vi "TstBldr_AnalysisScripts.vi"(0 "Engine reference":refnum<k7>, 1 "paths":T1, 2 "First call?":bool=TRUE, 5 "Sequence File Ref":refnum<k7>, 7 "Step Name":string="Run Script", 9 "Requirement":string, 11 "error in":errorcluster, 12 "Sequence index":i32, 13 "Conition Run?":bool, 14 "Attended?":bool) -> (3 "First call? out":bool, 4 "Engine reference (out)":refnum<k7>, 6 "Sequence File Ref(out)":refnum<k7>, 8 "Sequence index (out)":i32, 15 "error out":errorcluster)   [LabVIEW 2010]
doc: "This VI creates steps in TestStand for running analysis scripts in DIAdem"
uses:
  FilePaths.ctl
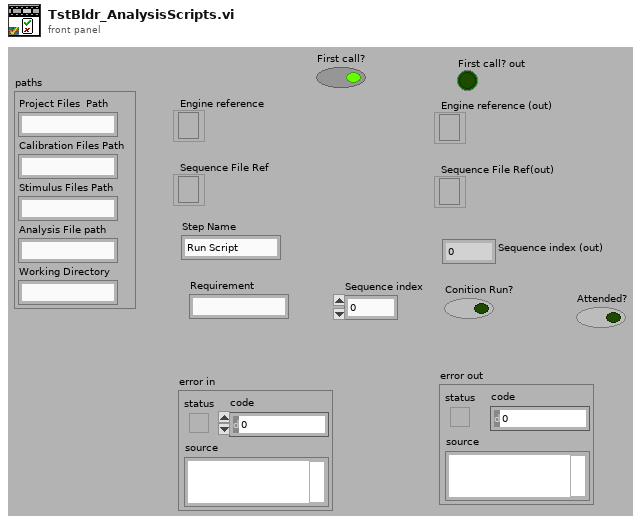
[diagram p1: front panel]
types:
  T1 = typedef "FilePaths.ctl" = cluster{"Project Files  Path":string, "Calibration Files Path":string, "Stimulus Files Path":string, "Analysis File path":string, "Working Directory":string}
  T2 = enum16{"Open DD Ref", "Export Paths", "Run Script", "Import Results", "Analysis Results", "Close DD Ref"}
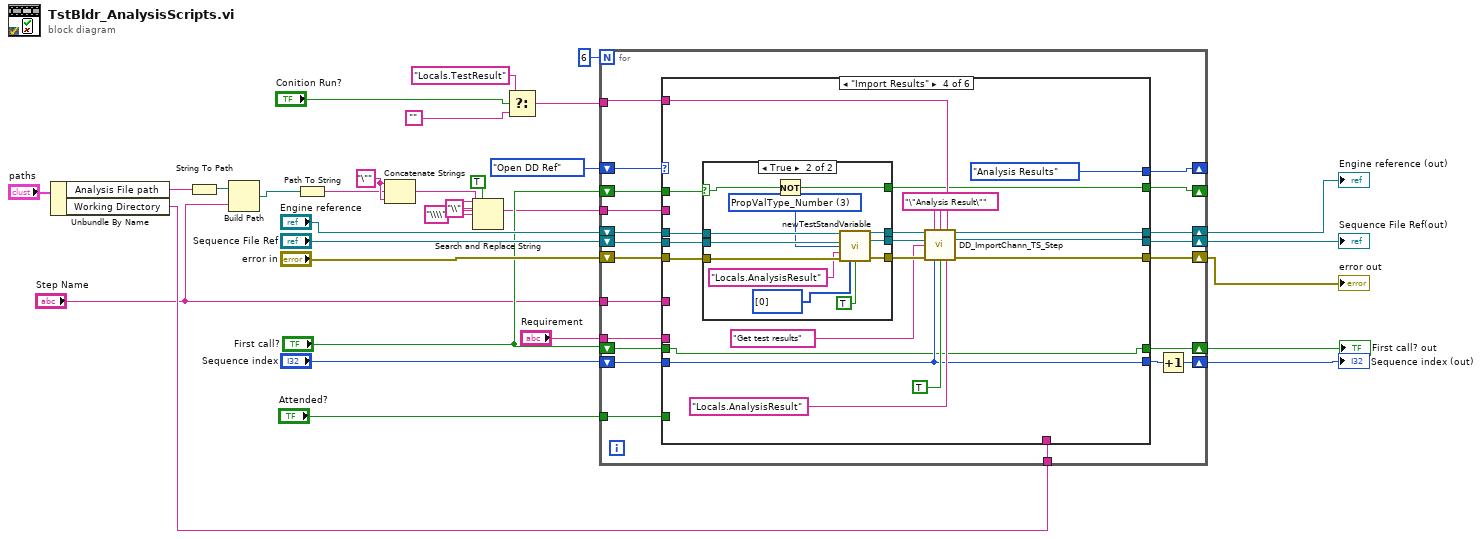
[diagram p0: block diagram]
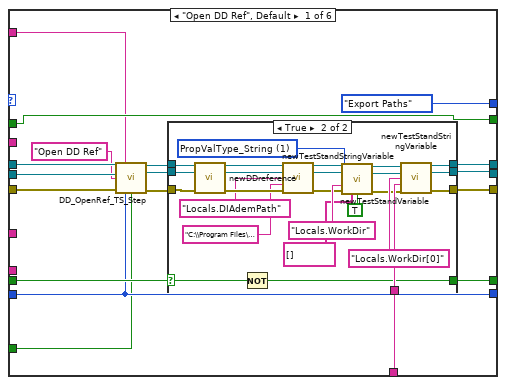
[diagram p2: hidden frame]
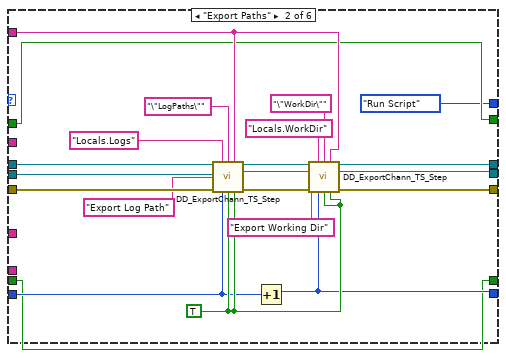
[diagram p4: hidden frame]
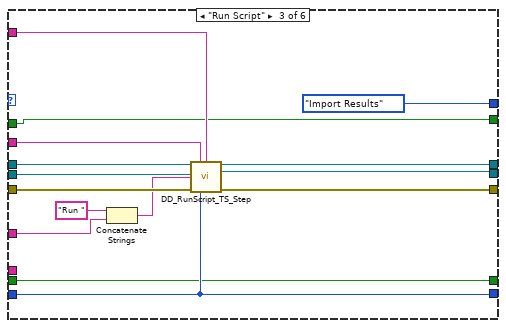
[diagram p5: hidden frame]
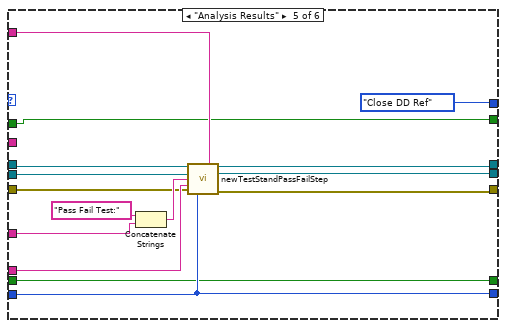
[diagram p7: hidden frame]
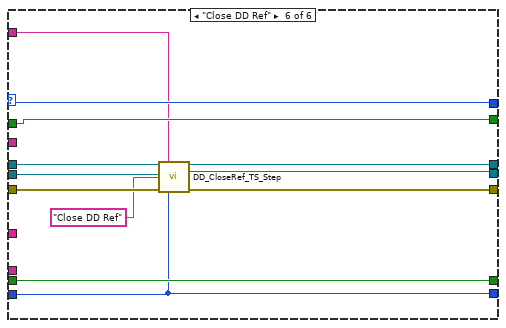
[diagram p8: hidden frame]
diagram:
  w11 = "\"" ("string")
  n1 = Unbundle By Name("paths") -> ("Analysis File path"=w5:string, "Working Directory"=w6:string)
  n2 = String To Path(string=w5) -> (path=w4:path)
  n3 = Build Path(base path=w4, name or relative path="Step Name") -> (appended path=w2:path)
  n4 = Path To String(path=w2) -> (string=w1:string)
  n5 = Concatenate Strings(w11, w1, w11) -> (w15:string)
  n6 = Search and Replace String(replace all?=TRUE ("replace all? (F)"), input string=w15, search string="\\", replace string="\\\\" ("replace string (\"\")")) -> (result string=w10:string)  [unwired: 4 in, 3 out]
  n7 = Select(t="Locals.TestResult", s="Conition Run?", f="") -> (s? t:f=w18:string)
  n8 = for {
    N: 6 -> [_]
    shift-right: [w48] -> w28
    shift-left: "Engine reference" -> [w51]
    shift-right: [w47] -> w29
    shift-left: "Sequence File Ref" -> [w50]
    shift-right: [w46] -> w30
    shift-left: "error in" -> [w49]
    shift-right: [w45] -> _
    shift-left: T2."Open DD Ref" -> [w52]
    tunnel: "Step Name" -> [w44]
    tunnel: w10 -> [w43]
    tunnel: "Requirement" -> [w41]
    tunnel: w6 -> [w40]
    shift-right: [w38] -> w31
    shift-left: "Sequence index" -> [w39]
    tunnel: w18 -> [w37]
    shift-right: [w35] -> w17
    shift-left: "First call?" -> [w36]
    shift-right: [w33] -> _
    shift-left: "First call?" -> [w34]
    tunnel: "Attended?" -> [w32]
    n9 = case shown="\"Import Results\"" w52 {
      selector: w52 -> [_ _ _ _ _ w188]
      tunnel: w51 -> [w60 w120 w135 w155 w186 w192]
      tunnel: w50 -> [w59 w119 w134 w154 w185 w191]
      tunnel: w49 -> [w63 w121 w136 w153 w172 w196]
      tunnel: [w70 w112 w132 w147 w184 w193] -> w48
      tunnel: [w69 w111 w130 w148 w183 w194] -> w47
      tunnel: [w68 w110 w131 w149 w182 w195] -> w46
      tunnel: [T2."Export Paths" T2."Run Script" T2."Import Results" T2."Analysis Results" T2."Close DD Ref" w188] -> w45
      tunnel: w39 -> [w58 w105 w129 w142 w181 w189]
      tunnel: w44 -> [_ _ w127 _ w178 _]
      tunnel: w43 -> [_ _ w133 _ _ _]
      tunnel: [w58 w104 w129 w142 w181 w189] -> w42
      tunnel: w41 -> [_ _ _ _ w180 _]
      tunnel: w40 -> [w67 _ _ _ _ _]
      tunnel: w37 -> [w53 w103 w125 w141 w176 w187]
      tunnel: w36 -> [w66 w102 w124 w140 w175 w198]
      tunnel: [w65 w102 w124 w140 w175 w198] -> w35
      tunnel: w34 -> [w64 w101 w123 w139 w174 w197]
      tunnel: [w64 w101 w123 w138 w174 w197] -> w33
      tunnel: w32 -> [w56 _ _ _ _ _]
      frame "Open DD Ref", Default {
        n10 = call "DD_OpenRef_TS_Step.vi"("Engine Reference"=w60, "Precondition"=w53, "Sequence File Ref"=w59, "Step Name"="Open DD Ref", "error in"=w63, "index"=w58, "Attended?"=w56) -> ("Engine reference(out)"=w62:refnum<k7>, "Sequence File Ref(out)"=w61:refnum<k7>, "error out"=w55:errorcluster)  [unwired: 6 in]
        n11 = case shown="True" w66 {
          selector: w66 -> [w71 w89]
          tunnel: w62 -> [w74 w85]
          tunnel: w61 -> [w73 w86]
          tunnel: w55 -> [w72 w87]
          tunnel: [w74 w99] -> w70
          tunnel: [w73 w98] -> w69
          tunnel: [w72 w97] -> w68
          tunnel: w67 -> [_ w95]
          tunnel: [w71 w88] -> w65
          frame False {
          }
          frame True {
            w91 = 1 items=["PropValType_Container", "PropValType_String", "PropValType_Boolean", "PropValType_Number", "PropValType_NamedType", "PropValType_Reference", "PropValType_Array"] ("Variable Type")
            n12 = call "newDDreference.vi"("Engine Reference"=w85, "Sequence File Ref"=w86, "error in"=w87) -> ("Engine Reference (out)"=w80:refnum<k7>, "Sequence File (out)"=w79:refnum<k7>, "error out"=w84:errorcluster)  [unwired: 10 in]
            n13 = Not(x=w89) -> (.not. x?=w88:bool)
            n14 = call "newTestStandStringVariable.vi"("Engine Reference"=w80, "Sequence File Ref"=w79, "Variable Name"="Locals.DIAdemPath", "Variable Value"="C:\\Program Files\\National Instruments\\DIAdem 11.1", "error in"=w84) -> ("Engine Reference (out)"=w82:refnum<k7>, "Sequence File (out)"=w81:refnum<k7>, "error out"=w83:errorcluster)  [unwired: 8 in]
            n15 = call "newTestStandVariable.vi"("Engine Reference"=w82, "Sequence File Ref"=w81, "Variable Type"=w91, "Variable Name"="Locals.WorkDir", "error in"=w83, "Variable Value"=string[] [], "Array?"=TRUE) -> ("Engine Reference(out)"=w93:refnum<k7>, "Sequence File Ref(out)"=w92:refnum<k7>, "error out"=w94:errorcluster)  [unwired: 6 in]
            n16 = call "newTestStandStringVariable.vi"("Engine Reference"=w93, "Sequence File Ref"=w92, "Variable Name"="Locals.WorkDir[0]", "Variable Value"=w95, "error in"=w94) -> ("Engine Reference (out)"=w99:refnum<k7>, "Sequence File (out)"=w98:refnum<k7>, "error out"=w97:errorcluster)  [unwired: 8 in]
          }
        }
      }
      frame "Export Paths" {
        w106 = TRUE ("Use Name?")
        n17 = call "DD_ExportChann_TS_Step.vi"("Engine Reference"=w120, "Source Data"="Locals.Logs", "Channel Name"="\"LogPaths\"", "Precondition"=w103, "Sequence File Ref"=w119, "Step Name"="Export Log Path", "error in"=w121, "index"=w105, "Use Name?"=w106, "CreateChannel?"=w106) -> ("Engine reference(out)"=w115:refnum<k7>, "Sequence File Ref(out)"=w113:refnum<k7>, "error out"=w114:errorcluster)  [unwired: 3 in]
        n18 = Increment(x=w105) -> (x+1=w104:i32)
        n19 = call "DD_ExportChann_TS_Step.vi"("Engine Reference"=w115, "Source Data"="Locals.WorkDir", "Channel Name"="\"WorkDir\"", "Precondition"=w103, "Sequence File Ref"=w113, "Step Name"="Export Working Dir", "error in"=w114, "index"=w104, "Use Name?"=w106, "CreateChannel?"=w106) -> ("Engine reference(out)"=w112:refnum<k7>, "Sequence File Ref(out)"=w111:refnum<k7>, "error out"=w110:errorcluster)  [unwired: 3 in]
      }
      frame "Run Script" {
        n20 = Concatenate Strings("Run " ("Step Name"), w127) -> (w126:string)
        n21 = call "DD_RunScript_TS_Step.vi"("Engine Reference"=w135, "Script Path"=w133, "Precondition"=w125, "Sequence File Ref"=w134, "Step Name"=w126, "error in"=w136, "index"=w129) -> ("Engine reference(out)"=w132:refnum<k7>, "Sequence File Ref(out)"=w130:refnum<k7>, "error out"=w131:errorcluster)  [unwired: 6 in]
      }
      frame "Import Results" {
        w145 = "\"Analysis Result\"" ("FirstChannel")
        n22 = case shown="True" w139 {
          selector: w139 -> [w156 w163]
          tunnel: w155 -> [w159 w171]
          tunnel: w154 -> [w158 w170]
          tunnel: w153 -> [w157 w169]
          tunnel: [w159 w166] -> w152
          tunnel: [w158 w165] -> w151
          tunnel: [w157 w164] -> w150
          tunnel: [w156 w162] -> w138
          frame False {
          }
          frame True {
            w168 = 3 items=["PropValType_Container", "PropValType_String", "PropValType_Boolean", "PropValType_Number", "PropValType_NamedType", "PropValType_Reference", "PropValType_Array"] ("Variable Type")
            n23 = Not(x=w163) -> (.not. x?=w162:bool)
            n24 = call "newTestStandVariable.vi"("Engine Reference"=w171, "Sequence File Ref"=w170, "Variable Type"=w168, "Variable Name"="Locals.AnalysisResult", "error in"=w169, "Variable Value"=i32[] [0], "Array?"=TRUE) -> ("Engine Reference(out)"=w166:refnum<k7>, "Sequence File Ref(out)"=w165:refnum<k7>, "error out"=w164:errorcluster)  [unwired: 6 in]
          }
        }
        n25 = call "DD_ImportChann_TS_Step.vi"("Engine Reference"=w152, "FirstChannel"=w145, "LastChannel"=w145, "Precondition"=w141, "Sequence File Ref"=w151, "Step Name"="Get test results", "error in"=w150, "index"=w142, "Use Name?"=TRUE, "Data Output"="Locals.AnalysisResult") -> ("Engine reference(out)"=w147:refnum<k7>, "Sequence File Ref(out)"=w148:refnum<k7>, "error out"=w149:errorcluster)  [unwired: 3 in]
      }
      frame "Analysis Results" {
        n26 = Concatenate Strings("Pass Fail Test:" ("Step Name"), w178) -> (w177:string)
        n27 = call "newTestStandPassFailStep.vi"("Engine Reference"=w186, "Precondition"=w176, "Sequence File Ref"=w185, "Step Name"=w177, "Requirement"=w180, "error in"=w172, "index"=w181) -> ("Engine reference(out)"=w184:refnum<k7>, "Sequence File Ref(out)"=w183:refnum<k7>, "error out"=w182:errorcluster)  [unwired: 6 in]
      }
      frame "Close DD Ref" {
        n28 = call "DD_CloseRef_TS_Step.vi"("Engine Reference"=w192, "Precondition"=w187, "Sequence File Ref"=w191, "Step Name"="Close DD Ref", "error in"=w196, "index"=w189) -> ("Engine reference(out)"=w193:refnum<k7>, "Sequence File Ref(out)"=w194:refnum<k7>, "error out"=w195:errorcluster)  [unwired: 7 in]
      }
    }
    n29 = Increment(x=w42) -> (x+1=w38:i32)
  }
  "Sequence index (out)" <- w31
  "error out" <- w30
  "Sequence File Ref(out)" <- w29
  "Engine reference (out)" <- w28
  "First call? out" <- w17
